vi "CFTS-Launcher.vi"() -> ()   [LabVIEW 2020]
uses:
  CFTS VIs/CFTS-Globals.vi
panel:
  out "Version":string
  out "Loading":string
  # "Cochlear Function Test Suite"
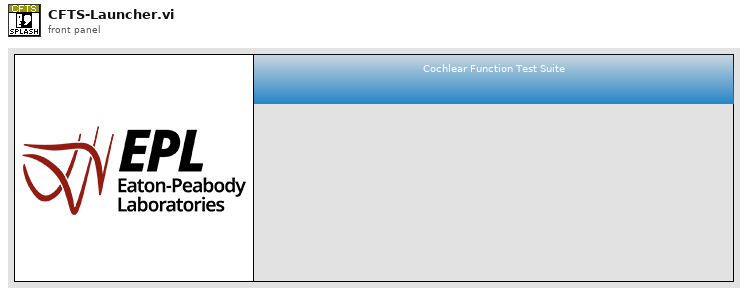
[diagram p1: front panel]
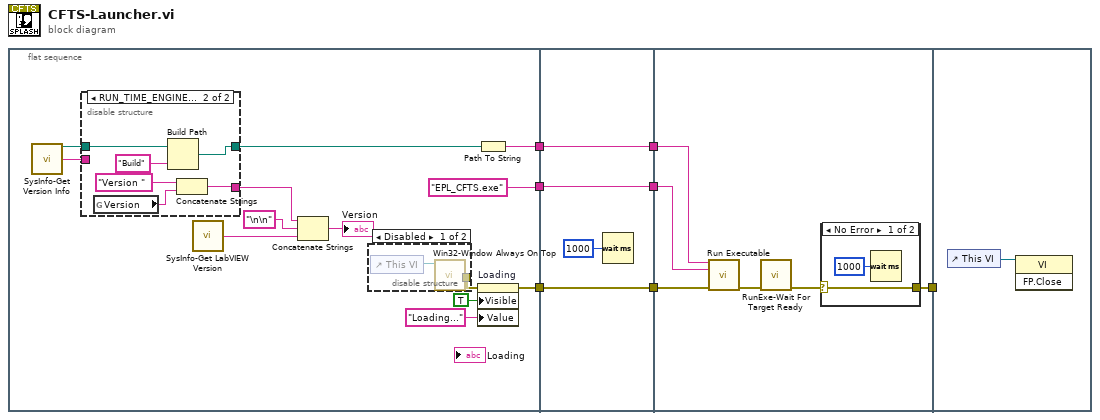
[diagram p0: block diagram]
diagram:
  n1 = flat-sequence {
    tunnel: [w18] -> w6
    tunnel: [w12] -> w4
    tunnel: ["EPL_CFTS.exe" (".EXE name")] -> w2
    tunnel: [w34] -> w7
    tunnel: w6 -> [w34]
    tunnel: [w33] -> w5
    tunnel: w4 -> [w33]
    tunnel: [w32] -> w3
    tunnel: w2 -> [w32]
    tunnel: w7 -> [w39]
    tunnel: w5 -> [w38]
    tunnel: w3 -> [w35]
    tunnel: [w37] -> w1
    tunnel: w1 -> [_]
    frame #0 {
      n2 = call "SysInfo-Get Version Info.vi"() -> ("folder"=w11:path, "formatted version"=w9:string)  [unwired: 13 in, 1 out]
      n3 = disable-structure shown="RUN_TIME_ENGINE==False, Default" {
        disable-tunnel: w11 -> [w24 w30]
        disable-tunnel: [w24 w28] -> w10
        disable-tunnel: w9 -> [w23 _]
        disable-tunnel: [w23 w25] -> w8
        frame condition #0 {
        }
        frame condition #1 (active) {
          n4 = global read "CFTS-Globals.vi" "Version"() -> (w27:string)
          n5 = Build Path(base path=w30, name or relative path="Build" ("Folder")) -> (appended path=w28:path)
          n6 = Concatenate Strings("Version ", w27) -> (w25:string)
        }
      }
      n7 = call "SysInfo-Get LabVIEW Version.vi"() -> ("Version Info"=w16:string)  [unwired: 15 in]
      n8 = Concatenate Strings(w8, "\n\n", w16) -> (→"Version":string)
      n9 = disable-structure shown="Disabled" {
        disable-tunnel: [w22 _] -> w17
        frame Disabled {
          n10 = control-ref of="This VI"() -> (w21:refnum<vi>)
          n11 = call "Win32-Window Always On Top.vi"("VI reference"=w21) -> ("error out"=w22:errorcluster)  [unwired: 9 in, 1 out]
        }
        frame Enabled {
        }
      }
      n12 = Path To String(path=w10) -> (string=w12:string)
      n13 = property on="Loading" class="Str"(error in=w17, "Visible"=TRUE, "Value"="Loading..." ("Loading")) -> (error out=w18:errorcluster)  [unwired: 1 in, 1 out]
    }
    frame #1 {
      n14 = Wait (ms)(milliseconds to wait=u32 1000) -> ()  [unwired: 1 out]
    }
    frame #2 {
      n15 = call "Run Executable.vi"("Folder"=w38, ".EXE name"=w35, "error in (no error)"=w39) -> ("error out"=w36:errorcluster)  [unwired: 12 in]
      n16 = call "RunExe-Wait For Target Ready.vi"("error in (no error)"=w36) -> ("error out"=w40:errorcluster)  [unwired: 14 in]
      n17 = case shown="No Error" w40 {
        selector: w40 -> [w41 w43]
        tunnel: [w41 w43] -> w37
        frame No Error {
          n18 = Wait (ms)(milliseconds to wait=u32 1000) -> ()  [unwired: 1 out]
        }
        frame Error {
        }
      }
    }
    frame #3 {
      n19 = control-ref of="This VI"() -> (w44:refnum<vi>)
      n20 = invoke class="VI" method="FP.Close"(reference=w44) -> ()  [unwired: 2 in, 3 out]
    }
  }
